vi "AG34980A_Configure_AC_Current.vi"(0 "VISA resource name":refnum<visa-resource-name>, 5 "Range (3:Auto)":T1(ring)=enum."Auto", 7 "Bandwidth (5:Default)":T2(ring)=enum."Default", 11 "error in (no error)":errorcluster) -> (4 "VISA resource name out":refnum<visa-resource-name>, 15 "error out":errorcluster)   [LabVIEW 2022 SP3, in "DMM_Keysight_34980A.lvlib" / "DMM_Keysight_34980A.lvclass"]
doc: "This VI allows you to control various settings for performing AC current measurements."
uses:
  DMM_Keysight_34980A.lvclass
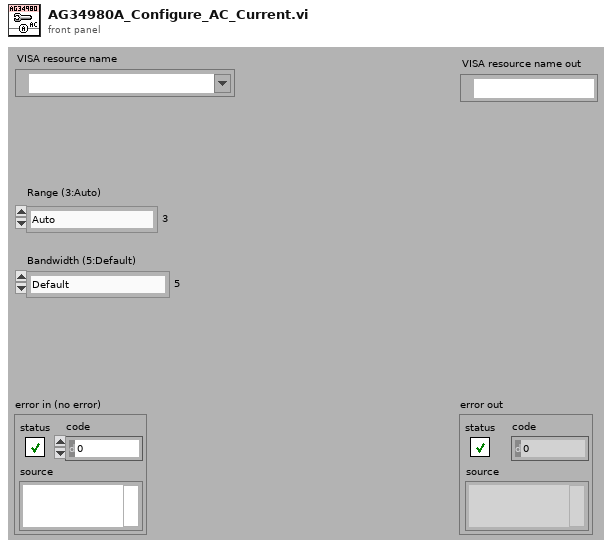
[diagram p1: front panel]
types:
  T1 = enum16{"10 mA", "100 mA", "1 A", "Auto", "Minimum", "Maximum", "Default"}
  T2 = enum16{"3 Hz", "20 Hz", "200 Hz", "Minimum", "Maximum", "Default"}
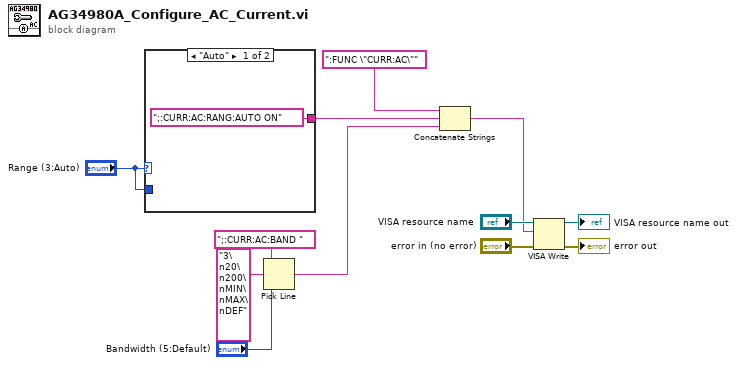
[diagram p0: block diagram]
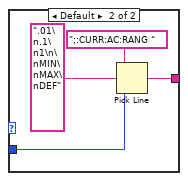
[diagram p2: hidden frame]
diagram:
  n1 = case shown="\"Auto\"" "Range (3:Auto)" {
    tunnel: [";:CURR:AC:RANG:AUTO ON" ("output string") w17] -> w7
    tunnel: "Range (3:Auto)" -> [_ w14]
    frame "Auto" {
    }
    frame Default {
      n2 = Pick Line(string ("")=";:CURR:AC:RANG ", multi-line string=".01\n.1\n1\n\nMIN\nMAX\nDEF", line index=w14) -> (output string=w17:string)
    }
  }
  n3 = Pick Line(string ("")=";:CURR:AC:BAND ", multi-line string="3\n20\n200\nMIN\nMAX\nDEF", line index="Bandwidth (5:Default)") -> (output string=w3:string)
  n4 = Concatenate Strings(":FUNC \"CURR:AC\"", w7, w3) -> (w8:string)
  n5 = VISA Write(VISA resource name="VISA resource name", write buffer=w8, error in (no error)="error in (no error)") -> (VISA resource name out=→"VISA resource name out":refnum<visa-resource-name>, error out=→"error out":errorcluster)  [unwired: 1 out]
